vi "NumeroAureo_Reciproco.vi"() -> (0 "Recíproco":dbl)   [LabVIEW 2022 SP3]
doc: "Determina el recíproco del número áureo: (sqrt(5)-1)/2"
panel:
  # "Numero aureo reciproco"
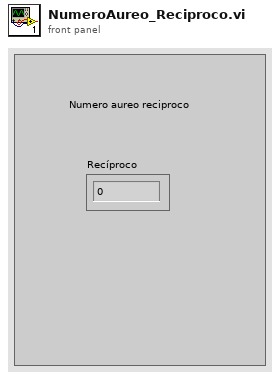
[diagram p1: front panel]
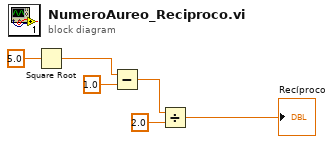
[diagram p0: block diagram]
diagram:
  n1 = Square Root(x=5.0) -> (sqrt(x)=w5:dbl)
  n2 = Subtract(x=w5, y=1.0) -> (x-y=w3:dbl)
  n3 = Divide(x=w3, y=2.0) -> (x/y=→"Recíproco":dbl)
